vi "Query Instrument.vi"(7 "Error Query (Enabled)":bool=TRUE caption="Error Query", 8 "error in":errorcluster, 10 "Command":string, 11 "VISA Resource Name":refnum<visa-resource-name>) -> (0 "error out":errorcluster, 2 "Response Strings":string[](array[string]), 3 "VISA Resource Name Out":refnum<visa-resource-name>)   [LabVIEW 2014, in "Hokuyo URG Series.lvlib"]
doc: "Performs the write of a command to the instrument, and reads the entire response string. This VI also checks the stats bit of the response for errors (if enabled) Different commands have different response structures, refer to the manual for information on each command."
uses:
  Hokuyo URG Series.lvlib
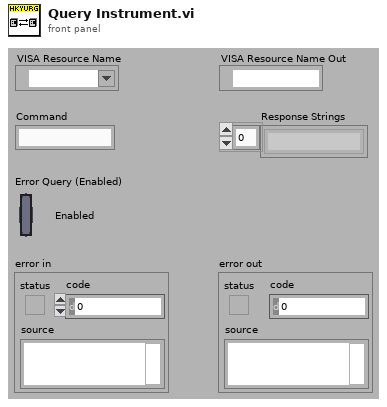
[diagram p1: front panel]
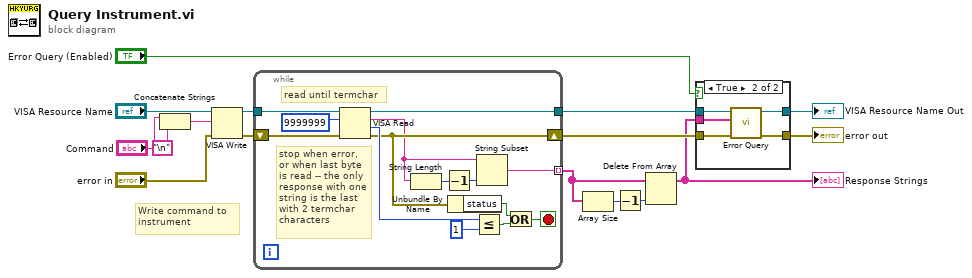
[diagram p0: block diagram]
diagram:
  # "Write command to\ninstrument"
  n1 = Concatenate Strings("Command", "\n") -> (w2:string)
  n2 = VISA Write(VISA resource name="VISA Resource Name", write buffer=w2, error in (no error)="error in") -> (VISA resource name out=w14:refnum<visa-resource-name>, error out=w13:errorcluster)  [unwired: 1 out]
  n3 = while {
    tunnel: w14 -> [w22]
    shift-right: [w23] -> w6
    shift-left: w13 -> [w25]
    tunnel: [w18] -> w10 mode=indexing
    tunnel: [w30] -> w8
    stop <- w27 stop-if-true
    # "stop when error, or when last byte is read -- the only response with one string is the last with 2 termchar characters"
    # "read until termchar"
    n4 = VISA Read(VISA resource name=w22, byte count=u32 9999999, error in (no error)=w25) -> (VISA resource name out=w30:refnum<visa-resource-name>, read buffer=w17:string, return count=w29:u32, error out=w23:errorcluster)
    n5 = String Length(string=w17) -> (length=w19:i32)
    n6 = Decrement(x=w19) -> (x-1=w20:i32)
    n7 = Unbundle By Name(w23) -> ("status"=w24:bool)
    n8 = Less Or Equal?(x=w29, y=u32 1) -> (x <= y?=w26:bool)
    n9 = String Subset(string=w17, length (rest)=w20) -> (substring=w18:string)  [unwired: 1 out]
    n10 = Or(x=w24, y=w26) -> (x .or. y?=w27:bool)
  }
  n11 = Array Size(array=w10) -> (size(s)=w12:i32)
  n12 = Decrement(x=w12) -> (x-1=w11:i32)
  n13 = Delete From Array(array=w10, index=w11) -> (array with subset deleted=w3:string[])  [unwired: 1 in, 1 out]
  "Response Strings" <- w3
  n14 = case shown="True" "Error Query (Enabled)" {
    tunnel: [w32 w36] -> w9
    tunnel: w8 -> [w32 w37]
    tunnel: w6 -> [w31 w35]
    tunnel: [w31 w34] -> w5
    tunnel: w3 -> [_ w33]
    frame False {
    }
    frame True {
      n15 = call "Error Query.vi"("error in (no error)"=w35, "Instrument Message"=w33, "VISA resource name"=w37) -> ("error out"=w34:errorcluster, "VISA resource out"=w36:refnum<visa-resource-name>)  [unwired: 5 in, 2 out]
    }
  }
  "error out" <- w5
  "VISA Resource Name Out" <- w9
